vi "GenTest1.vi"() -> ()   [LabVIEW 2020]
uses:
  <instrlib>/niFgen/niFgen.llb/niFgen_ctl Trigger SW - TrigName Values (Ring).ctl
  <instrlib>/niFgen/niFgen.llb/niFgen_ctl Trigger DigEdge - Edge Values (Ring).ctl
  <instrlib>/niFgen/niFgen.llb/niFgen_ctl Trigger DigLvl - Level Values (Ring).ctl
  <instrlib>/niFgen/niFgen.llb/niFgen_ctl Trigger Script - trigID Values (Ring).ctl
  <instrlib>/niFgen/niFgen.llb/niFgen Output Mode.ctl
  <instrlib>/niFgen/niFgen.llb/niFgen Configure Digital Edge Script Trigger.vi
  <instrlib>/niFgen/niFgen.llb/niFgen Disable Script Trigger.vi
  <instrlib>/niFgen/niFgen.llb/niFgen Write Named Waveform (I16).vi
  <instrlib>/niFgen/niFgen.llb/niFgen Configure Software Edge Script Trigger.vi
  <instrlib>/niFgen/niFgen.llb/niFgen Configure Digital Edge Start Trigger.vi
panel:
  in  "Resource Name":refnum<k15>="PXI1Slot2"
  in  "Script to Generate":u16(ring) items=["myScript0", "myScript1", "myScript2", "myScript3", "myScript4"]
  in  "Scripts Array":string[](array[string])=["script myScript0\n    Generate wfmSquare\n    Generate wfmSine\n    Generate wfmTriangle\n    Generate wfmSine\n    Generate wfmDC0V\nend script", "script myScript1\n  Wait until scriptTrigger0\n  Generate wfmSquare\n  Generate wfmSine\n  Generate wfmTriangle\n  Generate wfmSine\n  Generate wfmDC0V\nend script", "script myScript2\n  Generate wfmSquare\n  Repeat 2\n    Generate wfmSine\n  end repeat\n  Repeat 5\n    Generate wfmTriangle\n  end repeat\n  Repeat 2\n    Generate wfmSine\n  end repeat\n  Repeat 3\n    Generate wfmDC0V\n  end repeat\nend script", "script myScript3\n  Wait until scriptTrigger0\n  Generate wfmSquare\n  Repeat 2\n    Generate wfmSine\n  end repeat\n  Repeat 5\n    Generate wfmTriangle\n  end repeat\n  Repeat 2\n    Generate wfmSine\n  end repeat\n  Repeat 3\n    Generate wfmDC0V\n  end repeat\nend script", "script myScript4\n  Repeat forever\n    Generate wfmSquare\n    Repeat 2\n      Generate wfmSine\n    end repeat\n    Repeat 5\n      Generate wfmTriangle\n    end repeat\n    Repeat 2\n      Generate wfmSine\n    end repeat\n    Repeat 3\n      Generate wfmDC0V\n    end repeat\n  end repeat\nend script"]
  in  "Script Trigger Source":string(combo)="PFI1"
  in  "Waveform Information Array 2":T1(array[cluster])=[{"Name"="wfmSine", "Waveform"={"Waveform Type"=0, "Amplitude"=0.5, "# of points"=256}}, {"Name"="wfmSquare", "Waveform"={"Waveform Type"=3, "Amplitude"=1.0, "# of points"=256}}, {"Name"="wfmTriangle", "Waveform"={"Waveform Type"=2, "Amplitude"=0.5, "# of points"=256}}, {"Name"="wfmDC0V", "Waveform"={"Waveform Type"=7, "Amplitude"=0.0, "# of points"=256}}] caption="Waveform Information Array" {"Waveform"."Amplitude" min=0.0 max=1.0 format="%.2f"; "Waveform"."Waveform Type" items=["Sine", "Cosine", "Triangle", "Square", "Sawtooth", "Increasing Ramp", "Decreasing Ramp", "DC Value"]}
  in  "Script Trigger Type":u16(ring)=2 items=["None", "Software Edge", "Digital Edge", "Digital Level"]
  in  "FGEN Resource Name 2":refnum<k15> caption="FGEN Resource Name"
  in  "Stop 2":bool caption="Stop"
  in  "Send Software Trigger 2":bool caption="Send Software Trigger"
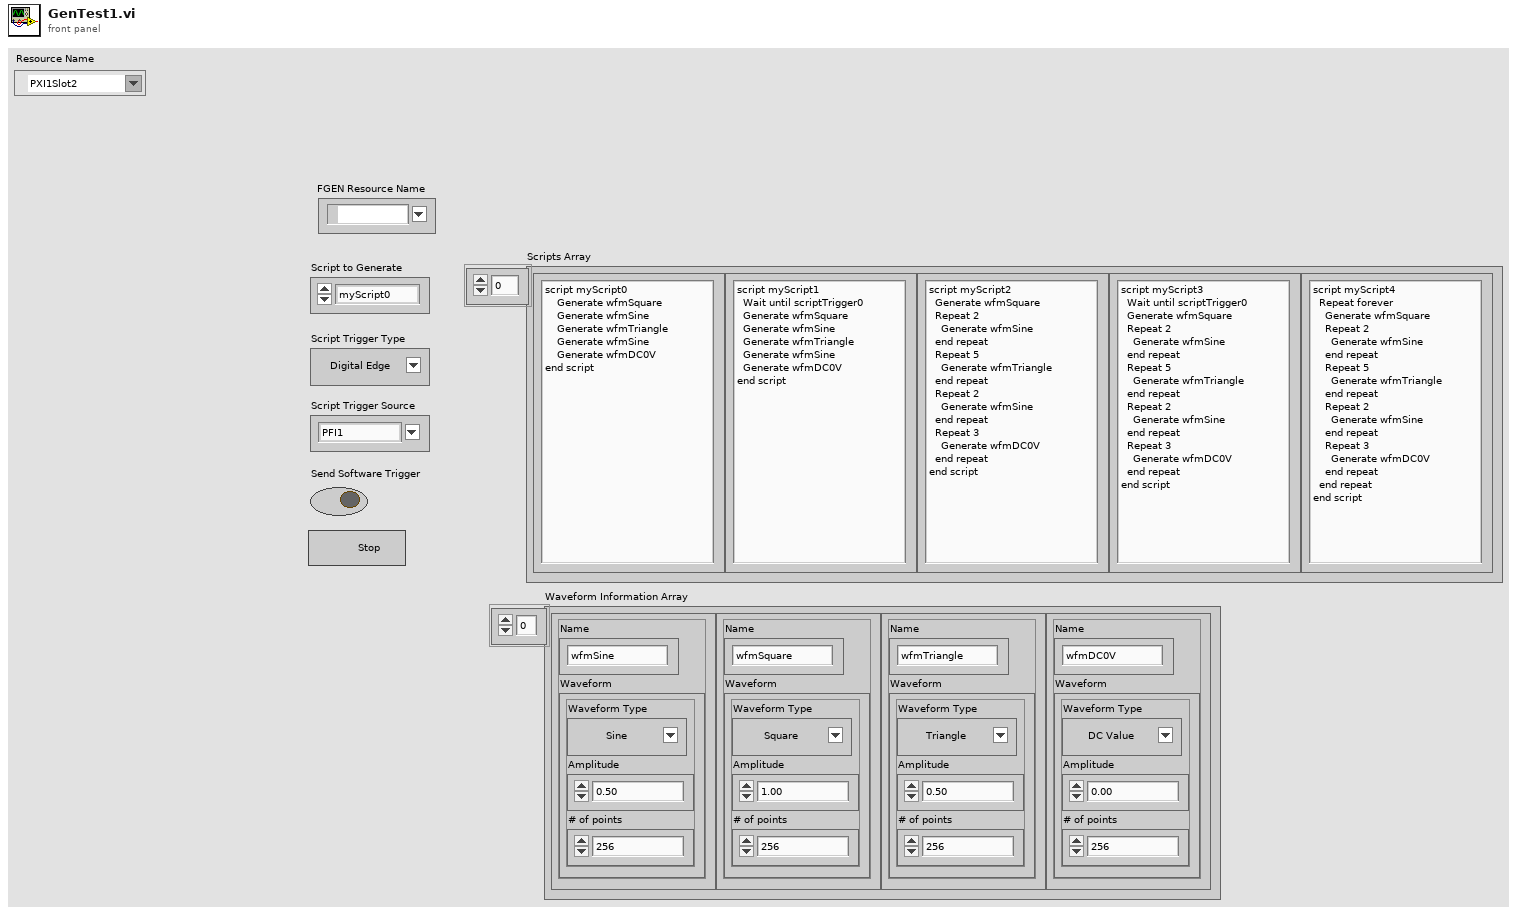
[diagram p1: front panel]
types:
  T1 = cluster{"Name":string, "Waveform":cluster{"Waveform Type":u16, "Amplitude":dbl, "# of points":u32}}[]
  T2 = typedef "niFgen Output Mode.ctl" = u32
  T3 = typedef "niFgen_ctl Trigger Script - trigID Values (Ring).ctl" = string
  T4 = typedef "niFgen_ctl Trigger DigEdge - Edge Values (Ring).ctl" = i32
  T5 = typedef "niFgen_ctl Trigger DigLvl - Level Values (Ring).ctl" = i32
  T6 = cluster{"Waveform Type":u16, "Amplitude":dbl, "# of points":u32}
  T7 = typedef "niFgen_ctl Trigger SW - TrigName Values (Ring).ctl" = i32
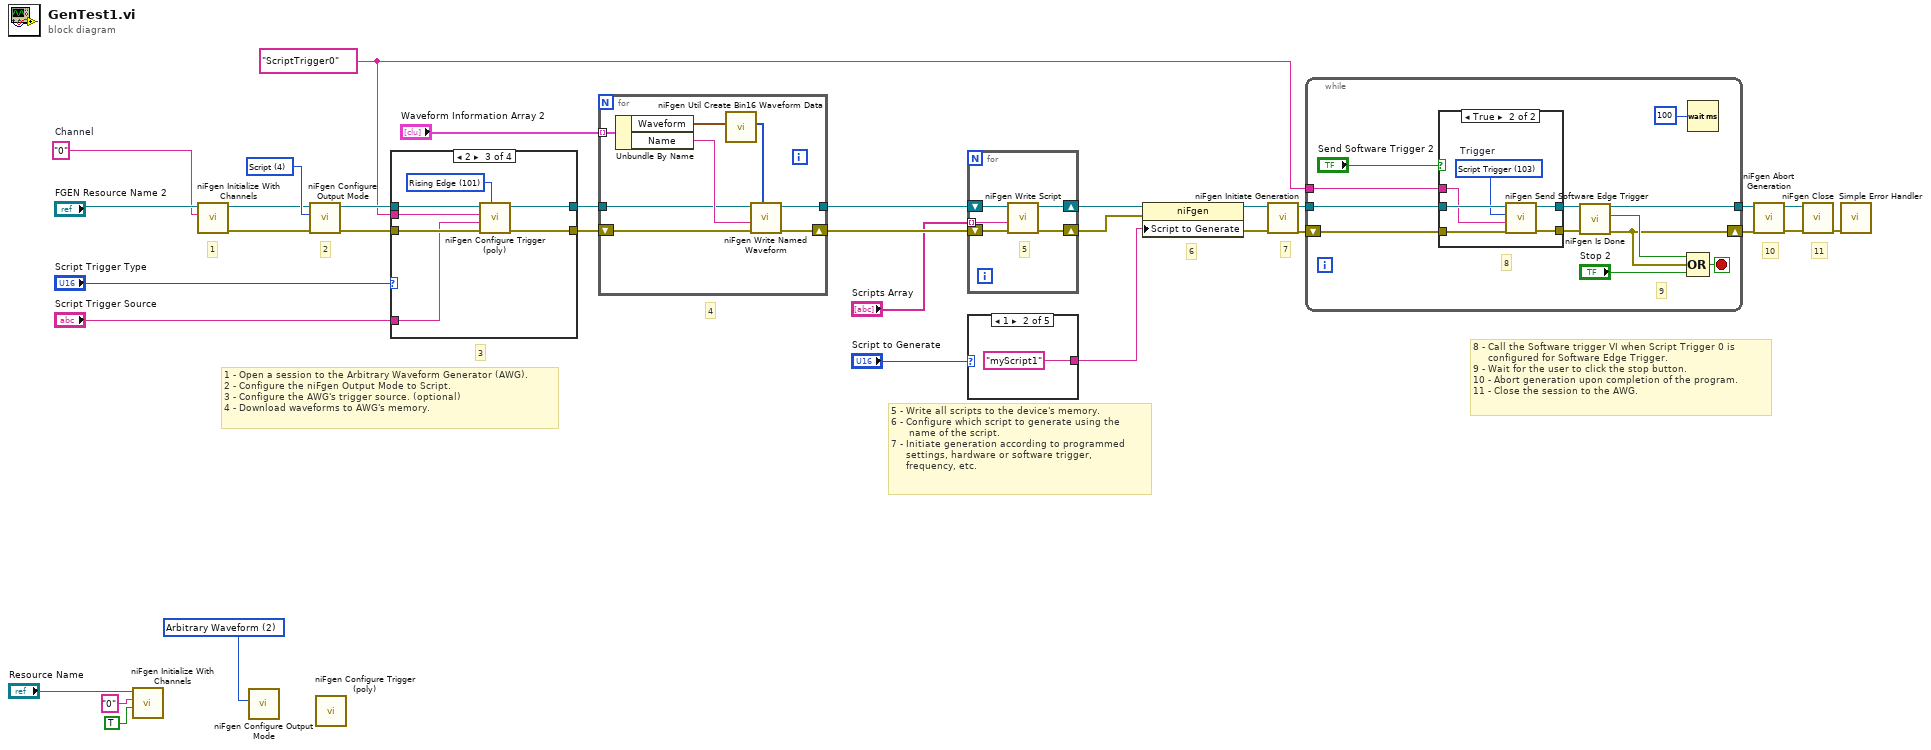
[diagram p0: block diagram]
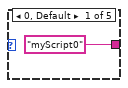
[diagram p2: hidden frame]
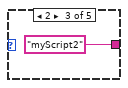
[diagram p3: hidden frame]
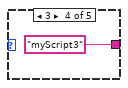
[diagram p4: hidden frame]
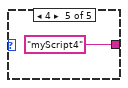
[diagram p5: hidden frame]
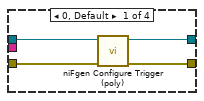
[diagram p6: hidden frame]
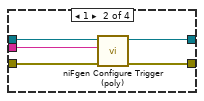
[diagram p7: hidden frame]
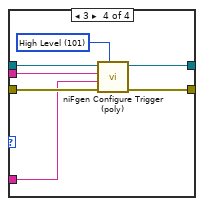
[diagram p8: hidden frame]
diagram:
  w3 = T2 2 items=["Standard Function", "Frequency List", "Arbitrary Waveform", "Arbitrary Sequence", "Script"] ("Output Mode (default: 0=Standard Function)")
  w7 = "0"  # Channel
  w21 = T2 4 items=["Standard Function", "Frequency List", "Arbitrary Waveform", "Arbitrary Sequence", "Script"] ("Output Mode")
  w25 = T3 "ScriptTrigger0" ("Trigger ID (Script Trigger 0)")
  # "6"
  # "11"
  # "10"
  # "7"
  # "4"
  # "3"
  # "2"
  # "1"
  # "8 - Call the Software trigger VI when Script Trigger 0 is \n     configured for Software Edge Trigger.\n9 - Wait for the user to click the stop button.\n10 - Abort generation upon completion of the program. \n11 - Close the session to the AWG."
  # "5 - Write all scripts to the device's memory.\n6 - Configure which script to generate using the \n      name of the script.\n7 - Initiate generation according to programmed \n     settings, hardware or software trigger, \n     frequency, etc."
  # "1 - Open a session to the Arbitrary Waveform Generator (AWG).\n2 - Configure the niFgen Output Mode to Script.\n3 - Configure the AWG's trigger source. (optional)\n4 - Download waveforms to AWG's memory."
  n1 = call <instrlib>:"niFgen Initialize With Channels.vi"("Reset Device (default: True)"=TRUE, "Channel Name"="0", "Resource Name"="Resource Name") -> ()  [unwired: 7 in, 2 out]
  n2 = call <instrlib>:"niFgen Initialize With Channels.vi"("Channel Name"=w7, "Resource Name"="FGEN Resource Name 2") -> ("error out"=w8:errorcluster, "Instrument Handle Out"=w9:refnum<k15>)  [unwired: 8 in]
  n3 = call <instrlib>:"niFgen Configure Output Mode.vi"("Output Mode (default: 0=Standard Function)"=w3) -> ("error in (no error)"=w1:errorcluster, "Instrument Handle"=w2:refnum<k15>)  [unwired: 6 in, 2 out]
  n4 = call <instrlib>:"niFgen Configure Output Mode.vi"("error in (no error)"=w8, "Output Mode (default: 0=Standard Function)"=w21, "Instrument Handle"=w9) -> ("error out"=w28:errorcluster, "Instrument Handle Out"=w29:refnum<k15>)  [unwired: 6 in]
  n5 = call-poly <instrlib>:"niFgen Configure Trigger (poly).vi"() -> ()  [unwired: 10 in, 2 out]
  n6 = case shown="2" "Script Trigger Type" {
    tunnel: w29 -> [w39 w44 w51 w58]
    tunnel: w28 -> [w38 w43 w50 w57]
    tunnel: [w37 w42 w49 w56] -> w27
    tunnel: [w36 w41 w48 w55] -> w26
    tunnel: w25 -> [_ w40 w47 w54]
    tunnel: "Script Trigger Source" -> [_ _ w45 w52]
    frame 0, Default {
      n7 = call-poly <instrlib>:"niFgen Configure Trigger (poly).vi"("error in (no error)"=w38, "Instrument Handle"=w39) -> ("error out"=w37:errorcluster, "Instrument Handle Out"=w36:refnum<k15>)  [unwired: 8 in]
    }
    frame 1 {
      n8 = call-poly <instrlib>:"niFgen Configure Trigger (poly).vi"("error in (no error)"=w43, "Trigger ID (Script Trigger 0)"=w40, "Instrument Handle"=w44) -> ("error out"=w42:errorcluster, "Instrument Handle Out"=w41:refnum<k15>)  [unwired: 7 in]
    }
    frame 2 {
      w46 = T4 101 items=["Rising Edge"=101, "Falling Edge"=102] ("Edge (Rising)")
      n9 = call-poly <instrlib>:"niFgen Configure Trigger (poly).vi"("Edge (Rising)"=w46, "error in (no error)"=w50, "Source"=w45, "Trigger ID (Script Trigger 0)"=w47, "Instrument Handle"=w51) -> ("error out"=w49:errorcluster, "Instrument Handle Out"=w48:refnum<k15>)  [unwired: 5 in]
    }
    frame 3 {
      w53 = T5 101 items=["High Level"=101, "Low Level"=102] ("Trigger When (High)")
      n10 = call-poly <instrlib>:"niFgen Configure Trigger (poly).vi"("Edge (Rising)"=w53, "error in (no error)"=w57, "Source"=w52, "Trigger ID (Script Trigger 0)"=w54, "Instrument Handle"=w58) -> ("error out"=w56:errorcluster, "Instrument Handle Out"=w55:refnum<k15>)  [unwired: 5 in]
    }
  }
  n11 = for {
    shift-right: [w63] -> w23
    shift-left: w27 -> [w61]
    tunnel: [w64] -> w24
    tunnel: w26 -> [w60]
    tunnel: "Waveform Information Array 2" -> [w66] mode=indexing
    n12 = Unbundle By Name(w66) -> ("Waveform"=w59:T6, "Name"=w62:string)
    n13 = call <instrlib>:"niFgen Util Create Bin16 Waveform Data.vi"("Waveform"=w59) -> ("Waveform Data"=w65:i16[])  [unwired: 10 in]
    n14 = call-poly <instrlib>:"niFgen Write Named Waveform.vi"("Waveform Data"=w65, "error in (no error)"=w61, "Waveform Name"=w62, "Instrument Handle"=w60) -> ("error out"=w63:errorcluster, "Instrument Handle Out"=w64:refnum<k15>)  [unwired: 5 in, 1 out]
  }
  n15 = for {
    shift-right: [w68] -> w15
    shift-left: w24 -> [w71]
    shift-right: [w69] -> w22
    shift-left: w23 -> [w70]
    tunnel: "Scripts Array" -> [w67] mode=indexing
    # "5"
    n16 = call <instrlib>:"niFgen Write Script.vi"("error in (no error)"=w70, "Script"=w67, "Instrument Handle"=w71) -> ("error out"=w69:errorcluster, "Instrument Handle Out"=w68:refnum<k15>)  [unwired: 7 in]
  }
  n17 = case shown="1" "Script to Generate" {
    tunnel: ["myScript0" "myScript1" "myScript2" "myScript3" "myScript4"] -> w11
    frame 0, Default {
    }
    frame 1 {
    }
    frame 2 {
    }
    frame 3 {
    }
    frame 4 {
    }
  }
  n18 = property class="niFgen"(reference=w15, error in=w22, "Script to Generate"=w11) -> (reference out=w14:refnum<k15>, error out=w16:errorcluster)
  n19 = call <instrlib>:"niFgen Initiate Generation.vi"("error in (no error)"=w16, "Instrument Handle"=w14) -> ("error out"=w32:errorcluster, "Instrument Handle Out"=w33:refnum<k15>)  [unwired: 8 in]
  n20 = while {
    tunnel: w33 -> [w88]
    tunnel: [w81] -> w31
    tunnel: w25 -> [w86]
    shift-right: [w77] -> w30
    shift-left: w32 -> [w87]
    stop <- w85 stop-if-true
    # "9"
    # "8"
    n21 = case shown="True" "Send Software Trigger 2" {
      tunnel: w88 -> [w90 w96]
      tunnel: w87 -> [w89 w95]
      tunnel: [w89 w94] -> w83
      tunnel: [w90 w93] -> w84
      tunnel: w86 -> [_ w91]
      frame False {
      }
      frame True {
        w92 = T7 103 items=["Start Trigger"=1004, "Script Trigger"=103]  # Trigger
        n22 = call <instrlib>:"niFgen Send Software Edge Trigger.vi"("error in (no error)"=w95, "Trigger ID (None)"=w91, "Trigger (Start Trigger)"=w92, "Instrument Handle"=w96) -> ("error out"=w94:errorcluster, "Instrument Handle Out"=w93:refnum<k15>)  [unwired: 6 in]
      }
    }
    n23 = call <instrlib>:"niFgen Is Done.vi"("error in (no error)"=w83, "Instrument Handle"=w84) -> ("error out"=w77:errorcluster, "Done"=w82:bool, "Instrument Handle Out"=w81:refnum<k15>)  [unwired: 7 in]
    n24 = Compound Arithmetic op=OR(w82, w77, "Stop 2") -> (w85:bool)
    n25 = Wait (ms)(milliseconds to wait=u32 100 ("millisecond multiple")) -> ()  [unwired: 1 out]
  }
  n26 = call <instrlib>:"niFgen Abort Generation.vi"("error in (no error)"=w30, "Instrument Handle"=w31) -> ("error out"=w34:errorcluster, "Instrument Handle Out"=w35:refnum<k15>)  [unwired: 8 in]
  n27 = call <instrlib>:"niFgen Close.vi"("error in (no error)"=w34, "Instrument Handle"=w35) -> ("error out"=w18:errorcluster)  [unwired: 9 in]
  n28 = call <vilib>:"Simple Error Handler.vi"("error in (no error)"=w18) -> ()  [unwired: 4 in, 5 out]
